vi "Read Current Parameter.vi"(8 "error in (no error)":errorcluster, 11 "AbstractExtractor in":refnum<class "AbstractExtractor.lvclass">) -> (0 "error out":errorcluster, 2 "AbstractData.lvclass":refnum<class "AbstractData.lvclass">, 3 "AbstractExtractor out":refnum<class "AbstractExtractor.lvclass">)   [LabVIEW 2014, in "AbstractExtractor.lvclass"]
uses:
  AbstractExtractor.lvclass
  Model/Data/AbstractData/AbstractData.lvclass
  AbstractExtractor.lvclass/AbstractExtractor.ctl
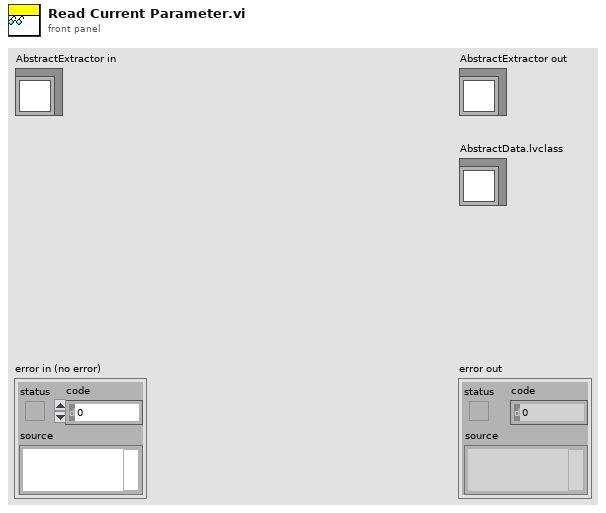
[diagram p1: front panel]
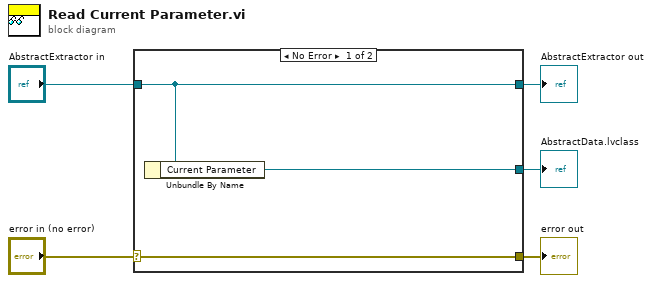
[diagram p0: block diagram]
diagram:
  n1 = case shown="No Error" "error in (no error)" {
    selector: "error in (no error)" -> [w8 w9]
    tunnel: [w8 w9] -> w4
    tunnel: [w7 w10] -> w2
    tunnel: "AbstractExtractor in" -> [w7 w10]
    tunnel: [w6 _] -> w1
    frame No Error {
      n2 = Unbundle By Name(w7) -> ("Current Parameter"=w6:refnum<class "AbstractData.lvclass">)
    }
    frame Error {
    }
  }
  "error out" <- w4
  "AbstractExtractor out" <- w2
  "AbstractData.lvclass" <- w1
